vi "Motor and Encoder (FPGA).vi"() -> ()   [LabVIEW 2016]
uses:
  <vilib>/Platform/TimedLoop/XDataNode/timing_clust.ctl
  <vilib>/Platform/TimedLoop/XDataNode/nitl_modes.ctl
  <vilib>/Platform/TimedLoop/XDataNode/wakeup.ctl
  <vilib>/rvi/Emulation/niFpgaSctlEmulationGetInTimedLoop.vi
  <vilib>/rvi/Emulation/niFpgaEmulationReportErrorSimple.vi
  <vilib>/rvi/Emulation/niFpgaGetClockAttributes.vi
  <vilib>/rvi/Emulation/niFpgaCriticalErrorInLSC.vi
  <vilib>/rvi/eio/common/nirviEmuTemplateMethod_errors.vi
  <vilib>/rvi/Emulation/niFpgaProcessEmulError.vi
  <vilib>/Platform/TimedLoop/XDataNode/XDataNode.xnode
  <vilib>/eio/EIONode/EIONode.xnode
  <vilib>/Platform/TimedLoop/XDataNode/XDNodeRunTimeDep.lvlib
panel:
  out "Index Pendulum Position":i32
  in  "Reset Pendulum Position Value":i32
  in  "Reset Pendulum Encoder Position":bool
  out "Pendulum Position":i32
  out "Pendulum Period Ticks":i32
  in  "Pendulum Direction Bit":bool
  out "Index Cart Position":i32
  in  "Reset Cart Position Value":i32
  in  "Reset Cart Encoder Position":bool
  out "Cart Position":i32
  out "Cart Period Ticks":i32
  in  "Cart Direction Bit":bool
  out "Index Fulcrum Position":i32
  in  "Reset Fulcrum Position Value":i32
  in  "Reset Fulcrum Encoder Position":bool
  out "Fulcrum Position":i32
  out "Fulcrum Period Ticks":i32
  in  "Cycles to Filter":u16=2
  in  "Fulcrum Direction Bit":bool
  in  "Duty Cycle Divisor":i16=2000
  in  "Duty Cycle (ticks)":i16
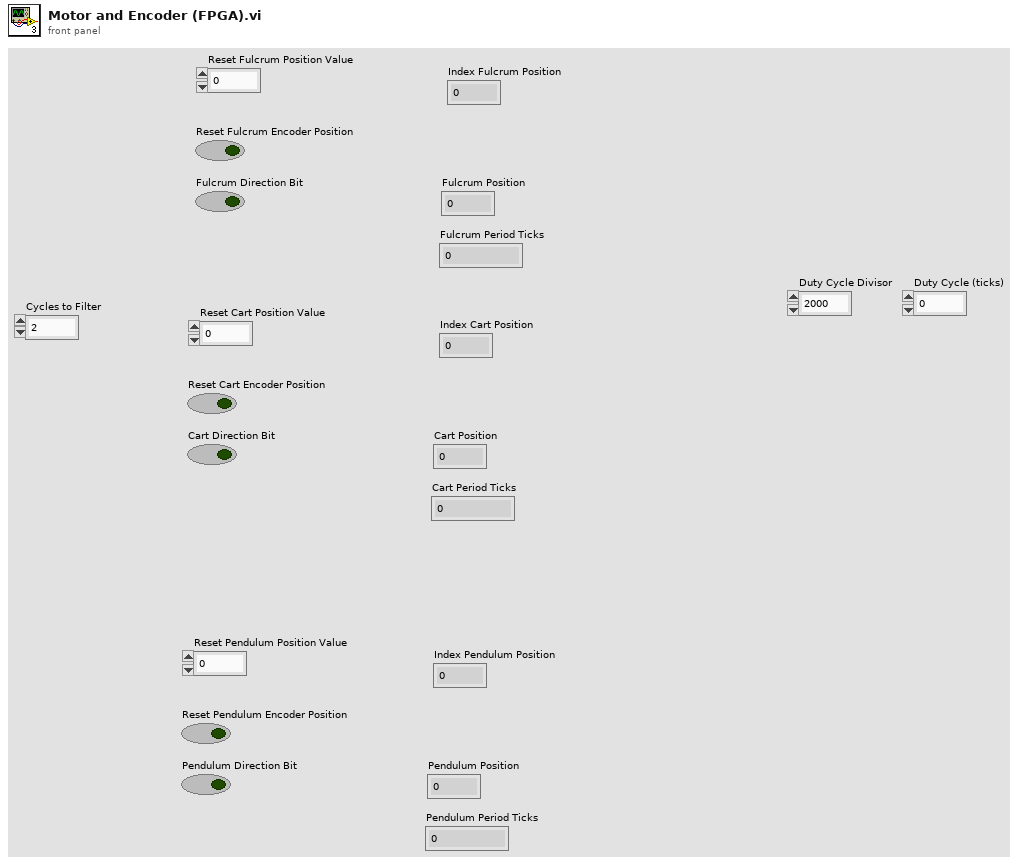
[diagram p1: front panel]
types:
  T1 = typedef "XDNodeRunTimeDep.lvlib/timing_clust.ctl" = cluster{"Expected End [f-1]":u64, "Actual End [f-1]":u64, "Finished Late? [f-1]":bool, "Expected End [i-1]":u64, "Actual End [i-1]":u64, "Finished Late? [i-1]":bool, "Expected Start [i]":u64, "Actual Start [i]":u64, "Expected Start [f]":u64, "Actual Start [f]":u64, "Source Name":string, "Structure Name":string, "Period":i64, "Deadline":i64, "Offset":i64, "Start":i64, "Priority":i32, "Timeout":i32, "Mode":T2, "Wakeup Reason":T3, "Error":errorcluster, "Source Type":string, "Secondary Source Type":string, "Global End Time":u64, "Global Start Time":u64, "Frame Duration":u64, "Iteration Duration":u64, "Assigned CPU":i32, "I/O Scan Engine Mode":u32}
  T2 = typedef "XDNodeRunTimeDep.lvlib/nitl_modes.ctl" = enum32{"No Change", "Process missed periods, maintain original phase", "Discard missed periods, maintain original phase", "Process missed periods, ignore original phase", "Discard missed periods, ignore original phase"}
  T3 = typedef "XDNodeRunTimeDep.lvlib/wakeup.ctl" = enum32{"Normal", "Aborted", "Asynchronous wakeup", "Timing source error", "Timed loop error", "Timeout"}
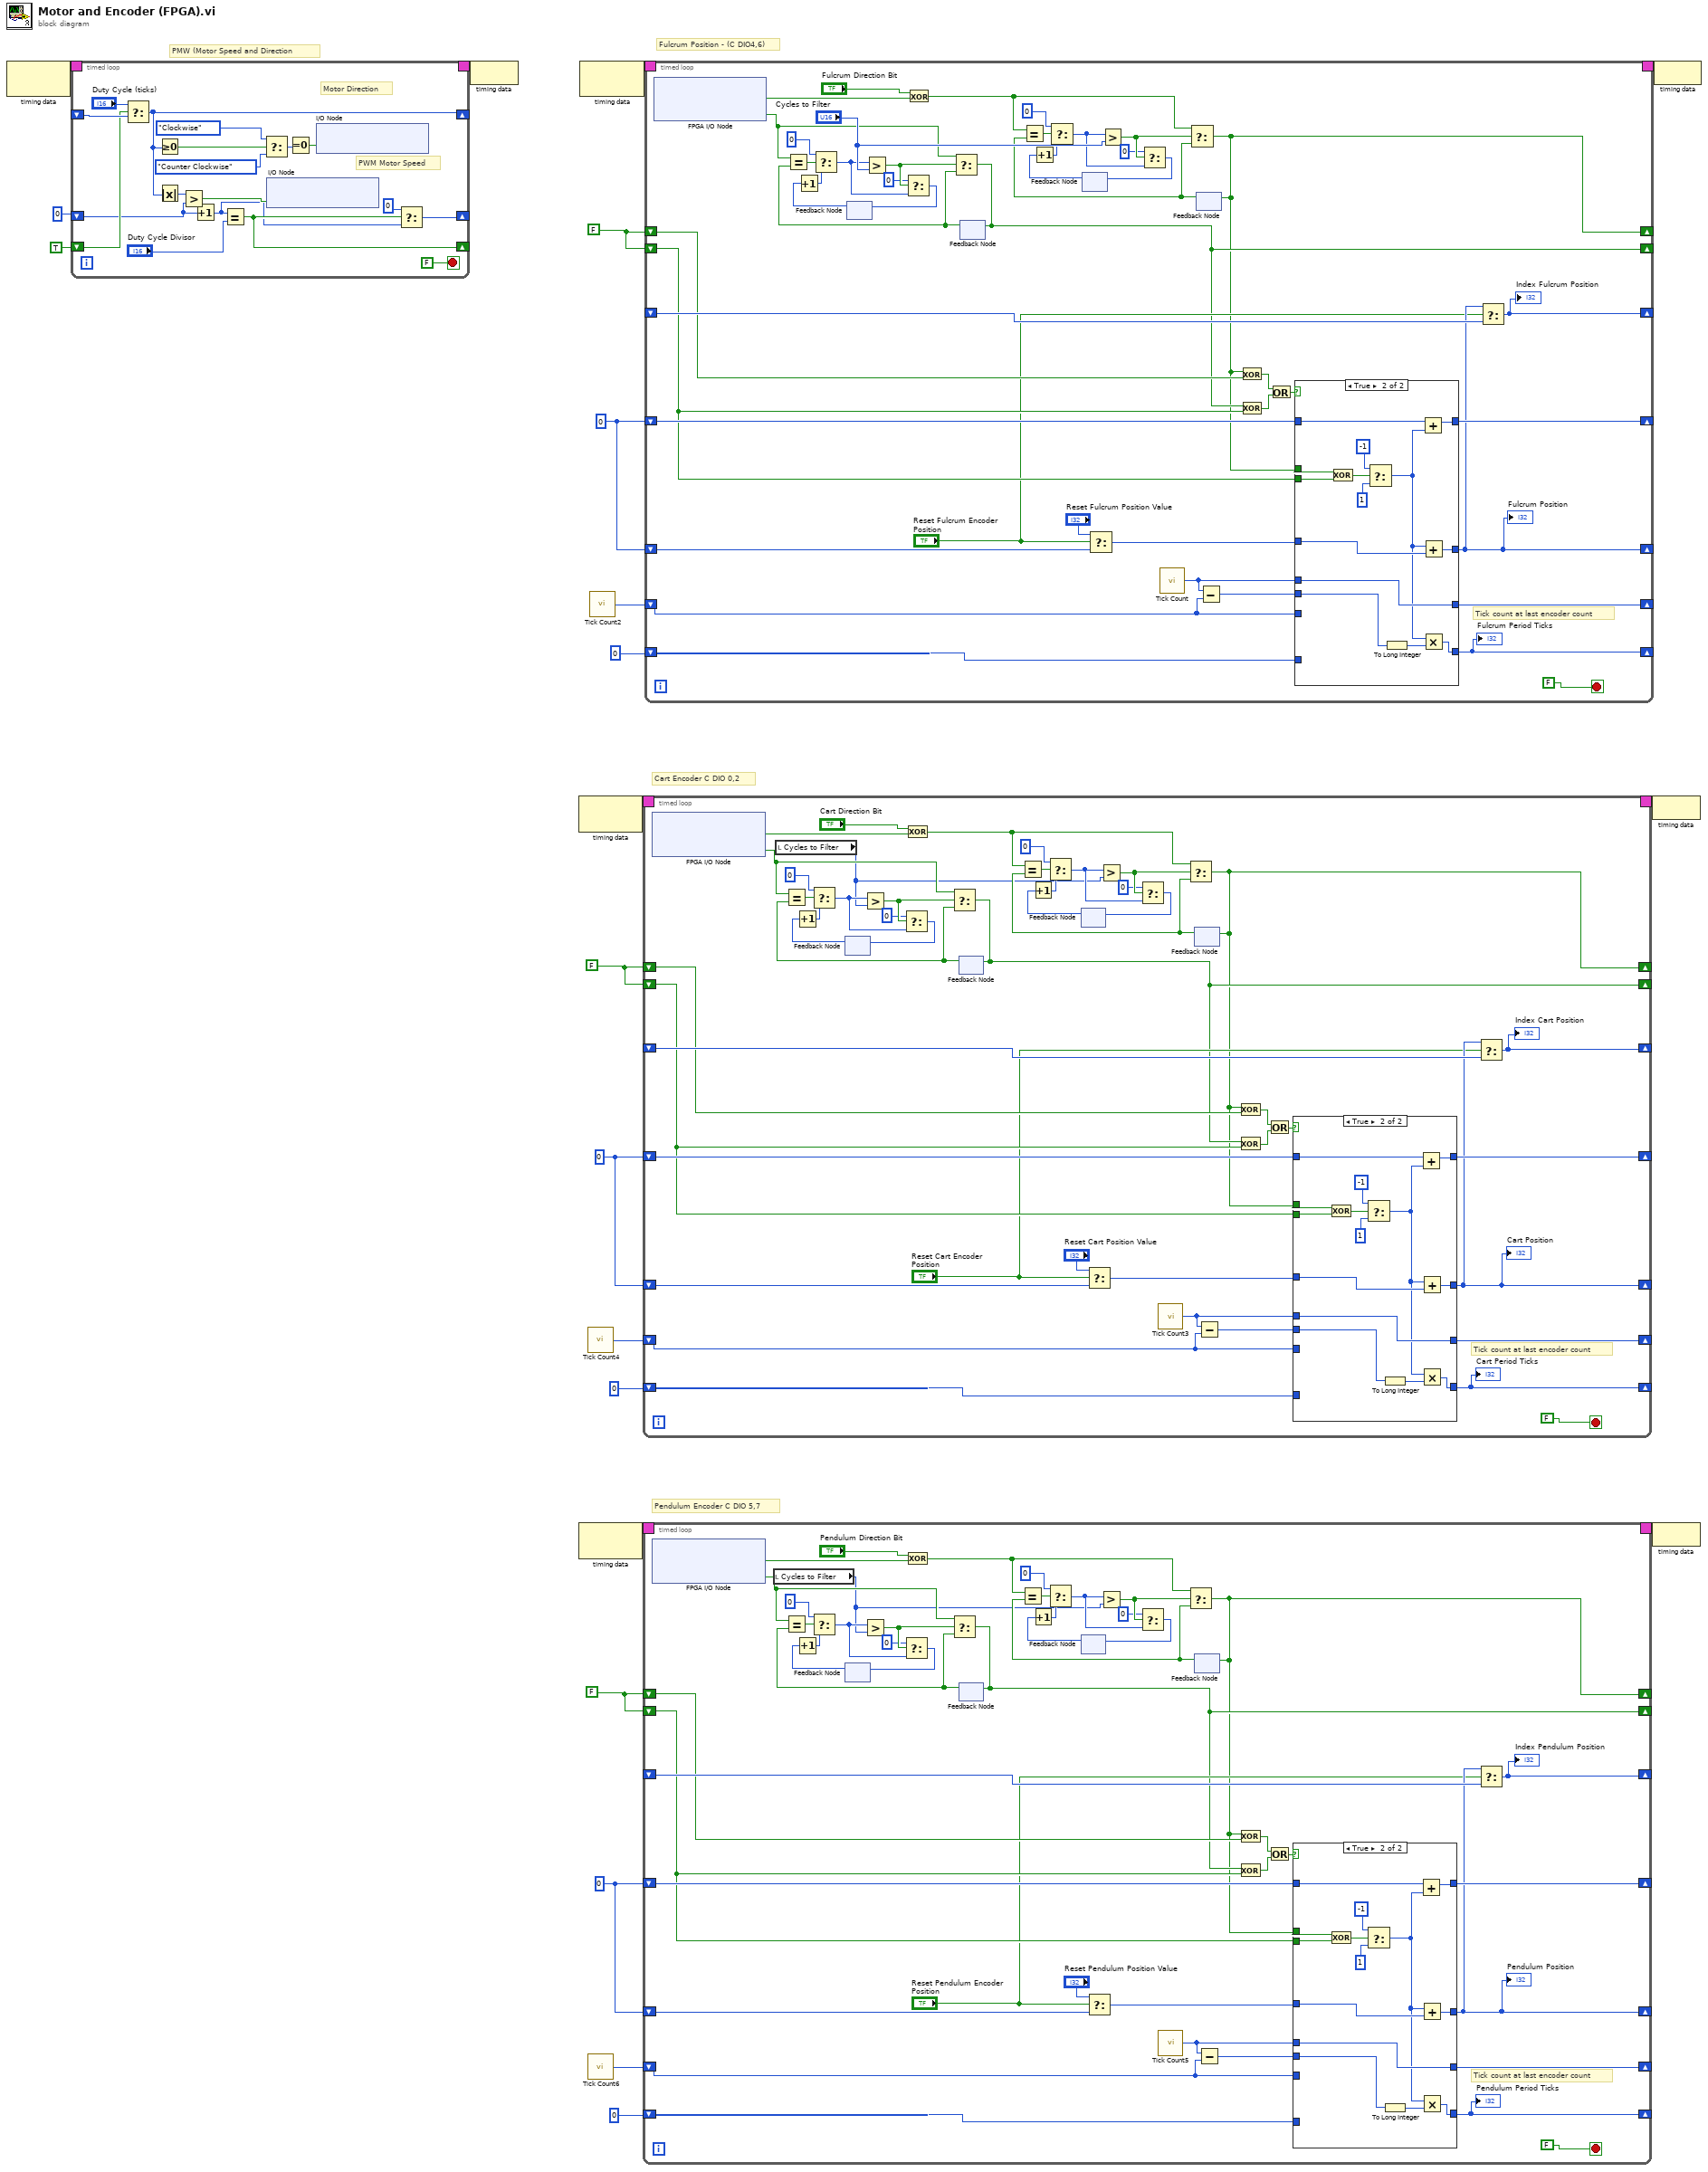
[diagram p0: block diagram]
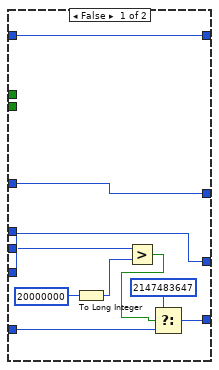
[diagram p2: hidden frame]
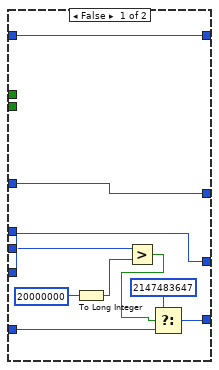
[diagram p3: hidden frame]
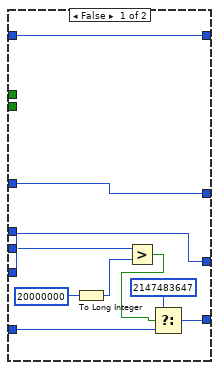
[diagram p4: hidden frame]
diagram:
  w3 = i16 0
  w4 = FALSE
  w9 = i16 0
  w10 = FALSE
  w15 = i16 0
  w16 = FALSE
  # "Pendulum Encoder C DIO 5,7"
  # "Cart Encoder C DIO 0,2"
  # "Fulcrum Position - (C DIO4,6)"
  # "PMW (Motor Speed and Direction"
  n1 = node-c288() -> (w22:T1)  [unwired: 1 in]
  n2 = timed-loop {
    timing: w22 -> [_]
    timing-out: [_] -> w21
    shift-right: [w32] -> _
    shift-left: _ -> [w39]
    shift-right: [w26] -> _
    shift-left: TRUE -> [w38]
    shift-right: [w28] -> _
    shift-left: i16 0 -> [w29]
    stop <- FALSE stop-if-true
    # "PWM Motor Speed"
    # "Motor Direction"
    n3 = Select(t="Duty Cycle (ticks)", s=w38, f=w39) -> (s? t:f=w32:i16)
    n4 = Greater Or Equal To 0?(x=w32) -> (x >= 0?=w37:bool)
    n5 = Absolute Value(x=w32) -> (abs(x)=w31:i16)
    n6 = Greater?(x=w31, y=w29) -> (0:w30:bool)
    n7 = Increment(x=w29) -> (x+1=w25:i16)
    n8 = Equal?(x=w25, y="Duty Cycle Divisor") -> (x = y?=w26:bool)
    n9 = Select(t=enum16{"Clockwise", "Counter Clockwise"}."Clockwise", s=w37, f=enum16{"Clockwise", "Counter Clockwise"}."Counter Clockwise") -> (s? t:f=w35:enum16{"Clockwise", "Counter Clockwise"})
    n10 = xnode "I/O Node"("ConnectorC/DIO3"=w30) -> ()  [unwired: 1 in, 1 out]
    n11 = Equal To 0?(x=w35) -> (x = 0?=w34:bool)
    n12 = xnode "I/O Node"("ConnectorC/DIO1"=w34) -> ()  [unwired: 1 in, 1 out]
    n13 = Select(t=i16 0, s=w26, f=w25) -> (s? t:f=w28:i16)
  }
  n14 = node-c288(w21) -> ()
  n15 = node-c288() -> (w12:T1)  [unwired: 1 in]
  n16 = node-c288() -> (w6:T1)  [unwired: 1 in]
  n17 = node-c288() -> (w18:T1)  [unwired: 1 in]
  n18 = call "Tick Count4"() -> ("Tick Count(Ticks)"=w8:u32)
  n19 = call "Tick Count6"() -> ("Tick Count(Ticks)"=w2:u32)
  n20 = call "Tick Count2"() -> ("Tick Count(Ticks)"=w14:u32)
  n21 = timed-loop {
    timing: w12 -> [_]
    timing-out: [_] -> w11
    shift-right: [w48] -> _
    shift-left: w10 -> [w83]
    shift-right: [w49] -> _
    shift-left: w10 -> [w81]
    shift-right: [w88] -> _
    shift-left: _ -> [w87]
    shift-right: [w80] -> _
    shift-left: w9 -> [w82]
    shift-right: [w76] -> _
    shift-left: w9 -> [w78]
    shift-right: [w75] -> _
    shift-left: w8 -> [w72]
    shift-right: [w70] -> _
    shift-left: i16 0 -> [w71]
    stop <- FALSE stop-if-true
    # "Tick count at last encoder count"
    n22 = xnode "FPGA I/O Node"() -> ("ConnectorC/DIO0"=w46:bool, "ConnectorC/DIO2"=w47:bool)  [unwired: 2 in, 2 out]
    n23 = local read "Cycles to Filter"() -> (w43:u16)
    n24 = feedback #1() -> (w58:u16)  [unwired: 1 out]
    n25 = Increment(x=w58) -> (x+1=w54:u16)
    n26 = Exclusive Or(1:w46, 2:"Cart Direction Bit") -> (0:w45:bool)
    n27 = feedback #2() -> (w56:bool)  [unwired: 1 out]
    n28 = Equal?(x=w47, y=w56) -> (x = y?=w57:bool)
    n29 = Select(t=u16 0 ("f"), s=w57, f=w54) -> (s? t:f=w51:u16)
    n30 = Greater?(x=w51, y=w43) -> (0:w53:bool)
    n31 = Select(t=u16 0, s=w53, f=w51) -> (s? t:f=w52:u16)
    n32 = feedback-in #1(w52) -> ()
    n33 = Select(t=w47, s=w53, f=w56) -> (s? t:f=w49:bool)
    n34 = feedback-in #2(w49) -> ()
    n35 = feedback #3() -> (w67:u16)  [unwired: 1 out]
    n36 = Increment(x=w67) -> (x+1=w63:u16)
    n37 = Select(t="Reset Cart Position Value", s="Reset Cart Encoder Position", f=w78) -> (s? t:f=w77:i32)
    n38 = call "Tick Count3"() -> ("Tick Count(Ticks)"=w74:u32)
    n39 = feedback #4() -> (w65:bool)  [unwired: 1 out]
    n40 = Equal?(x=w45, y=w65) -> (x = y?=w66:bool)
    n41 = Select(t=u16 0 ("f"), s=w66, f=w63) -> (s? t:f=w60:u16)
    n42 = Greater?(x=w60, y=w43) -> (0:w62:bool)
    n43 = Select(t=u16 0, s=w62, f=w60) -> (s? t:f=w61:u16)
    n44 = feedback-in #3(w61) -> ()
    n45 = Select(t=w45, s=w62, f=w65) -> (s? t:f=w48:bool)
    n46 = feedback-in #4(w48) -> ()
    n47 = Subtract(x=w74, y=w72) -> (x-y=w73:u32)
    n48 = Exclusive Or(1:w83, 2:w48) -> (0:w85:bool)
    n49 = Exclusive Or(1:w81, 2:w49) -> (0:w84:bool)
    n50 = Or(x=w85, y=w84) -> (x .or. y?=w86:bool)
    n51 = case shown="True" w86 {
      tunnel: w82 -> [w98 w111]
      tunnel: [w98 w112] -> w80
      tunnel: w48 -> [_ w110]
      tunnel: w81 -> [_ w109]
      tunnel: w77 -> [w97 w106]
      tunnel: [w97 w107] -> w76
      tunnel: w74 -> [_ w103]
      tunnel: [w96 w103] -> w75
      tunnel: w73 -> [w95 w100]
      tunnel: w72 -> [w96 _]
      tunnel: w71 -> [w90 _]
      tunnel: [w89 w99] -> w70
      frame False {
        n52 = To Long Integer(number=20000000) -> (32bit integer=w93:i32)
        n53 = Greater?(x=w95, y=w93) -> (0:w91:bool)
        n54 = Select(t=2147483647, s=w91, f=w90) -> (s? t:f=w89:i32)
      }
      frame True {
        n55 = Exclusive Or(1:w109, 2:w110) -> (0:w108:bool)
        n56 = Select(t=i16 -1, s=w108, f=i16 1) -> (s? t:f=w102:i16)
        n57 = To Long Integer(number=w100) -> (32bit integer=w101:i32)
        n58 = Add(x=w111, y=w102) -> (x+y=w112:i16)
        n59 = Add(x=w102, y=w106) -> (x+y=w107:i32)
        n60 = Multiply(x=w102, y=w101) -> (x*y=w99:i32)
      }
    }
    "Cart Position" <- w76
    "Cart Period Ticks" <- w70
    n61 = Select(t=w76, s="Reset Cart Encoder Position", f=w87) -> (s? t:f=w88:i32)
    "Index Cart Position" <- w88
  }
  n62 = timed-loop {
    timing: w6 -> [_]
    timing-out: [_] -> w5
    shift-right: [w120] -> _
    shift-left: w4 -> [w155]
    shift-right: [w121] -> _
    shift-left: w4 -> [w153]
    shift-right: [w160] -> _
    shift-left: _ -> [w159]
    shift-right: [w152] -> _
    shift-left: w3 -> [w154]
    shift-right: [w148] -> _
    shift-left: w3 -> [w150]
    shift-right: [w147] -> _
    shift-left: w2 -> [w144]
    shift-right: [w142] -> _
    shift-left: i16 0 -> [w143]
    stop <- FALSE stop-if-true
    # "Tick count at last encoder count"
    n63 = xnode "FPGA I/O Node"() -> ("ConnectorC/DIO5"=w118:bool, "ConnectorC/DIO7"=w119:bool)  [unwired: 2 in, 2 out]
    n64 = local read "Cycles to Filter"() -> (w115:u16)
    n65 = feedback #5() -> (w130:u16)  [unwired: 1 out]
    n66 = Increment(x=w130) -> (x+1=w126:u16)
    n67 = Exclusive Or(1:w118, 2:"Pendulum Direction Bit") -> (0:w117:bool)
    n68 = feedback #6() -> (w128:bool)  [unwired: 1 out]
    n69 = Equal?(x=w119, y=w128) -> (x = y?=w129:bool)
    n70 = Select(t=u16 0 ("f"), s=w129, f=w126) -> (s? t:f=w123:u16)
    n71 = Greater?(x=w123, y=w115) -> (0:w125:bool)
    n72 = Select(t=u16 0, s=w125, f=w123) -> (s? t:f=w124:u16)
    n73 = feedback-in #5(w124) -> ()
    n74 = Select(t=w119, s=w125, f=w128) -> (s? t:f=w121:bool)
    n75 = feedback-in #6(w121) -> ()
    n76 = feedback #7() -> (w139:u16)  [unwired: 1 out]
    n77 = Increment(x=w139) -> (x+1=w135:u16)
    n78 = Select(t="Reset Pendulum Position Value", s="Reset Pendulum Encoder Position", f=w150) -> (s? t:f=w149:i32)
    n79 = call "Tick Count5"() -> ("Tick Count(Ticks)"=w146:u32)
    n80 = feedback #8() -> (w137:bool)  [unwired: 1 out]
    n81 = Equal?(x=w117, y=w137) -> (x = y?=w138:bool)
    n82 = Select(t=u16 0 ("f"), s=w138, f=w135) -> (s? t:f=w132:u16)
    n83 = Greater?(x=w132, y=w115) -> (0:w134:bool)
    n84 = Select(t=u16 0, s=w134, f=w132) -> (s? t:f=w133:u16)
    n85 = feedback-in #7(w133) -> ()
    n86 = Select(t=w117, s=w134, f=w137) -> (s? t:f=w120:bool)
    n87 = feedback-in #8(w120) -> ()
    n88 = Subtract(x=w146, y=w144) -> (x-y=w145:u32)
    n89 = Exclusive Or(1:w155, 2:w120) -> (0:w157:bool)
    n90 = Exclusive Or(1:w153, 2:w121) -> (0:w156:bool)
    n91 = Or(x=w157, y=w156) -> (x .or. y?=w158:bool)
    n92 = case shown="True" w158 {
      tunnel: w154 -> [w170 w183]
      tunnel: [w170 w184] -> w152
      tunnel: w120 -> [_ w182]
      tunnel: w153 -> [_ w181]
      tunnel: w149 -> [w169 w178]
      tunnel: [w169 w179] -> w148
      tunnel: w146 -> [_ w175]
      tunnel: [w168 w175] -> w147
      tunnel: w145 -> [w167 w172]
      tunnel: w144 -> [w168 _]
      tunnel: w143 -> [w162 _]
      tunnel: [w161 w171] -> w142
      frame False {
        n93 = To Long Integer(number=20000000) -> (32bit integer=w165:i32)
        n94 = Greater?(x=w167, y=w165) -> (0:w163:bool)
        n95 = Select(t=2147483647, s=w163, f=w162) -> (s? t:f=w161:i32)
      }
      frame True {
        n96 = Exclusive Or(1:w181, 2:w182) -> (0:w180:bool)
        n97 = Select(t=i16 -1, s=w180, f=i16 1) -> (s? t:f=w174:i16)
        n98 = To Long Integer(number=w172) -> (32bit integer=w173:i32)
        n99 = Add(x=w183, y=w174) -> (x+y=w184:i16)
        n100 = Add(x=w174, y=w178) -> (x+y=w179:i32)
        n101 = Multiply(x=w174, y=w173) -> (x*y=w171:i32)
      }
    }
    "Pendulum Position" <- w148
    "Pendulum Period Ticks" <- w142
    n102 = Select(t=w148, s="Reset Pendulum Encoder Position", f=w159) -> (s? t:f=w160:i32)
    "Index Pendulum Position" <- w160
  }
  n103 = timed-loop {
    timing: w18 -> [_]
    timing-out: [_] -> w17
    shift-right: [w191] -> _
    shift-left: w16 -> [w227]
    shift-right: [w192] -> _
    shift-left: w16 -> [w225]
    shift-right: [w232] -> _
    shift-left: _ -> [w231]
    shift-right: [w224] -> _
    shift-left: w15 -> [w226]
    shift-right: [w220] -> _
    shift-left: w15 -> [w222]
    shift-right: [w219] -> _
    shift-left: w14 -> [w216]
    shift-right: [w214] -> _
    shift-left: i16 0 -> [w215]
    stop <- FALSE stop-if-true
    # "Tick count at last encoder count"
    n104 = xnode "FPGA I/O Node"() -> ("ConnectorC/DIO4"=w189:bool, "ConnectorC/DIO6"=w190:bool)  [unwired: 2 in, 2 out]
    n105 = feedback #9() -> (w201:u16)  [unwired: 1 out]
    n106 = Increment(x=w201) -> (x+1=w197:u16)
    n107 = Exclusive Or(1:w189, 2:"Fulcrum Direction Bit") -> (0:w188:bool)
    n108 = feedback #10() -> (w199:bool)  [unwired: 1 out]
    n109 = Equal?(x=w190, y=w199) -> (x = y?=w200:bool)
    n110 = Select(t=u16 0 ("f"), s=w200, f=w197) -> (s? t:f=w194:u16)
    n111 = Greater?(x=w194, y="Cycles to Filter") -> (0:w196:bool)
    n112 = Select(t=u16 0, s=w196, f=w194) -> (s? t:f=w195:u16)
    n113 = feedback-in #9(w195) -> ()
    n114 = Select(t=w190, s=w196, f=w199) -> (s? t:f=w192:bool)
    n115 = feedback-in #10(w192) -> ()
    n116 = feedback #11() -> (w210:u16)  [unwired: 1 out]
    n117 = Increment(x=w210) -> (x+1=w206:u16)
    n118 = Select(t="Reset Fulcrum Position Value", s="Reset Fulcrum Encoder Position", f=w222) -> (s? t:f=w221:i32)
    n119 = call "Tick Count"() -> ("Tick Count(Ticks)"=w218:u32)
    n120 = feedback #12() -> (w208:bool)  [unwired: 1 out]
    n121 = Equal?(x=w188, y=w208) -> (x = y?=w209:bool)
    n122 = Select(t=u16 0 ("f"), s=w209, f=w206) -> (s? t:f=w203:u16)
    n123 = Greater?(x=w203, y="Cycles to Filter") -> (0:w205:bool)
    n124 = Select(t=u16 0, s=w205, f=w203) -> (s? t:f=w204:u16)
    n125 = feedback-in #11(w204) -> ()
    n126 = Select(t=w188, s=w205, f=w208) -> (s? t:f=w191:bool)
    n127 = feedback-in #12(w191) -> ()
    n128 = Subtract(x=w218, y=w216) -> (x-y=w217:u32)
    n129 = Exclusive Or(1:w227, 2:w191) -> (0:w229:bool)
    n130 = Exclusive Or(1:w225, 2:w192) -> (0:w228:bool)
    n131 = Or(x=w229, y=w228) -> (x .or. y?=w230:bool)
    n132 = case shown="True" w230 {
      tunnel: w226 -> [w242 w255]
      tunnel: [w242 w256] -> w224
      tunnel: w191 -> [_ w254]
      tunnel: w225 -> [_ w253]
      tunnel: w221 -> [w241 w250]
      tunnel: [w241 w251] -> w220
      tunnel: w218 -> [_ w247]
      tunnel: [w240 w247] -> w219
      tunnel: w217 -> [w239 w244]
      tunnel: w216 -> [w240 _]
      tunnel: w215 -> [w234 _]
      tunnel: [w233 w243] -> w214
      frame False {
        n133 = To Long Integer(number=20000000) -> (32bit integer=w237:i32)
        n134 = Greater?(x=w239, y=w237) -> (0:w235:bool)
        n135 = Select(t=2147483647, s=w235, f=w234) -> (s? t:f=w233:i32)
      }
      frame True {
        n136 = Exclusive Or(1:w253, 2:w254) -> (0:w252:bool)
        n137 = Select(t=i16 -1, s=w252, f=i16 1) -> (s? t:f=w246:i16)
        n138 = To Long Integer(number=w244) -> (32bit integer=w245:i32)
        n139 = Add(x=w255, y=w246) -> (x+y=w256:i16)
        n140 = Add(x=w246, y=w250) -> (x+y=w251:i32)
        n141 = Multiply(x=w246, y=w245) -> (x*y=w243:i32)
      }
    }
    "Fulcrum Position" <- w220
    "Fulcrum Period Ticks" <- w214
    n142 = Select(t=w220, s="Reset Fulcrum Encoder Position", f=w231) -> (s? t:f=w232:i32)
    "Index Fulcrum Position" <- w232
  }
  n143 = node-c288(w11) -> ()
  n144 = node-c288(w5) -> ()
  n145 = node-c288(w17) -> ()
